vi "CPP_FFTBoost.vi"(5 "CutoffFrequency":dbl=200.0, 7 "MaxBoost":dbl=15.0, 8 "dF":dbl, 9 "UnwrappedPhaseLag":dbl[](array[numeric]), 10 "AmplitudeBoost":dbl[](array[numeric]), 11 "Muffleddata":dbl[](array[numeric])) -> (1 "BandLimitedBoost":dbl[](array[numeric]), 3 "boostedData":dbl[](array[numeric]), 4 "CutoffFrequencyUsed":dbl=15.0, 6 "MaxBoostUsed":dbl=15.0)   [LabVIEW 2011]
uses:
  <vilib>/Analysis/2dsp.llb/Real FFT.vi
  <vilib>/Analysis/2dsp.llb/Inverse Real FFT.vi
  <vilib>/Analysis/NI_AALPro.lvlib
panel:
  in  "PhaseCorrection":bool=TRUE
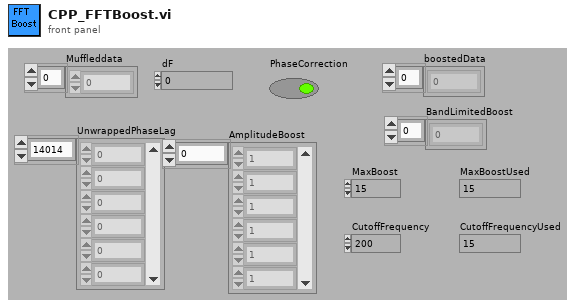
[diagram p1: front panel]
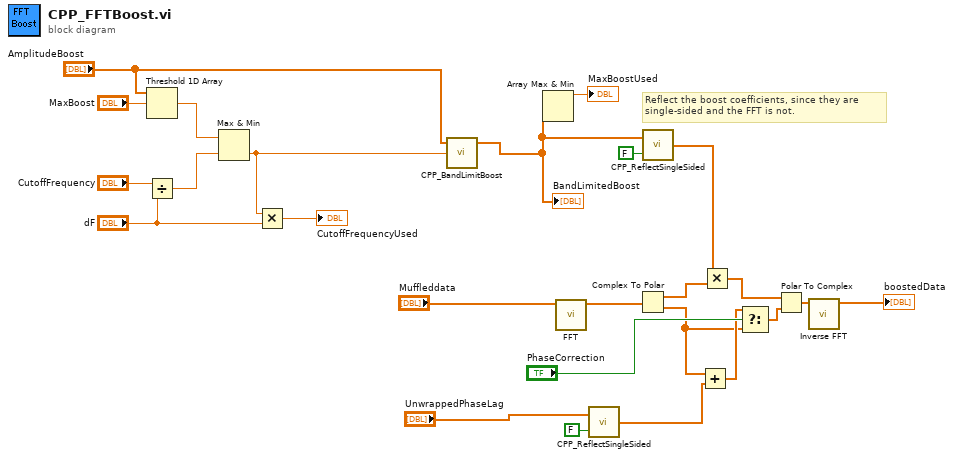
[diagram p0: block diagram]
diagram:
  # "Reflect the boost coefficients, since they are single-sided and the FFT is not."
  n1 = Threshold 1D Array(2:"MaxBoost", 3:"AmplitudeBoost") -> (0:w15:dbl)  [unwired: 1 in]
  n2 = Divide(x="CutoffFrequency", y="dF") -> (x/y=w16:dbl)
  n3 = Max & Min(x=w15, y=w16) -> (min(x,y)=w12:dbl)  [unwired: 1 out]
  n4 = Multiply(x=w12, y="dF") -> (x*y=→"CutoffFrequencyUsed":dbl)
  n5 = call "CPP_BandLimitBoost.vi"("CutoffIndex"=w12, "AmplitudeBoost"="AmplitudeBoost") -> ("Filtered X"=w1:dbl[])  [unwired: 2 in, 1 out]
  "BandLimitedBoost" <- w1
  n6 = Array Max & Min(array=w1) -> (max value=→"MaxBoostUsed":dbl)  [unwired: 3 out]
  n7 = call-poly <vilib>:"FFT.vi"("X"="Muffleddata") -> ("FFT {X}"=w21:cdb[])  [unwired: 9 in, 1 out]
  n8 = call "CPP_ReflectSingleSided.vi"("DC Present?"=FALSE, "SingleSidedData"="UnwrappedPhaseLag") -> ("DCandReflectedData"=w19:dbl[])
  n9 = Complex To Polar(r * e^(i*theta)=w21) -> (r=w22:dbl[], theta=w4:dbl[])
  n10 = call "CPP_ReflectSingleSided.vi"("DC Present?"=FALSE, "SingleSidedData"=w1) -> ("DCandReflectedData"=w11:dbl[])
  n11 = Add(x=w4, y=w19) -> (x+y=w6:dbl[])
  n12 = Multiply(x=w11, y=w22) -> (x*y=w23:dbl[])
  n13 = Select(t=w6, s="PhaseCorrection", f=w4) -> (s? t:f=w5:dbl[])
  n14 = Polar To Complex(1:w5, 2:w23) -> (0:w24:cdb[])
  n15 = call-poly <vilib>:"Inverse FFT.vi"("FFT {X}"=w24) -> ("X"=→"boostedData":dbl[])  [unwired: 9 in, 1 out]
